vi "MaxIntenProj.vi"(10 "Dimension":u16, 11 "3D Array":u16[][][](array[numeric])) -> (3 "MaxProj":u16[][](array[numeric]))   [LabVIEW 2015]
panel:
  out "Intensity Graph":u16[][](graph)
  out "before size":i32[](array[numeric])
  out "size(s)":i32[](array[numeric])
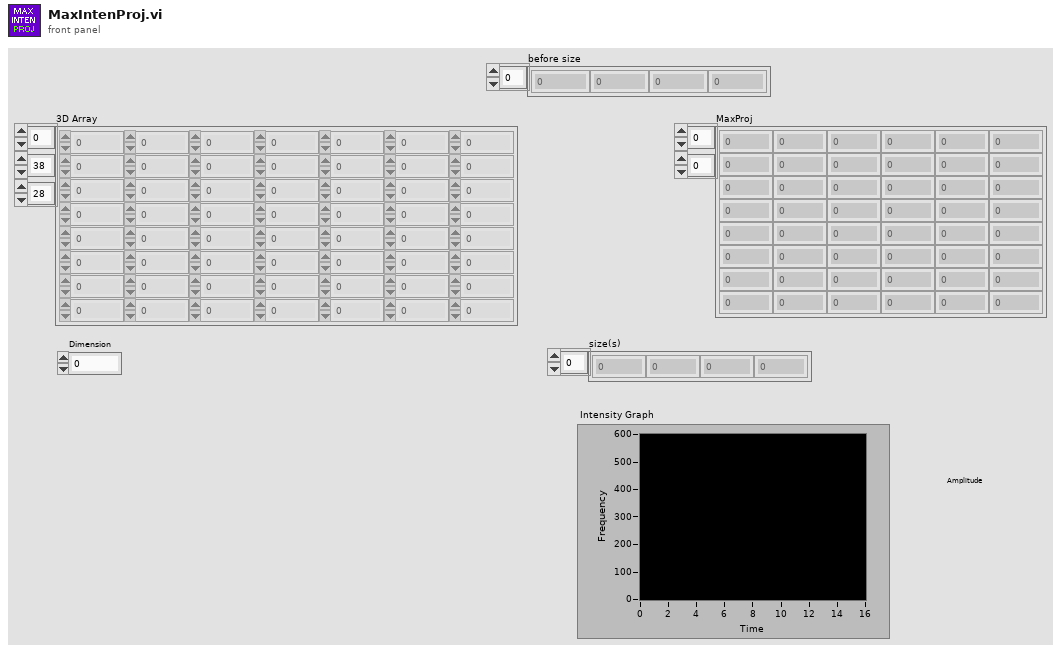
[diagram p1: front panel]
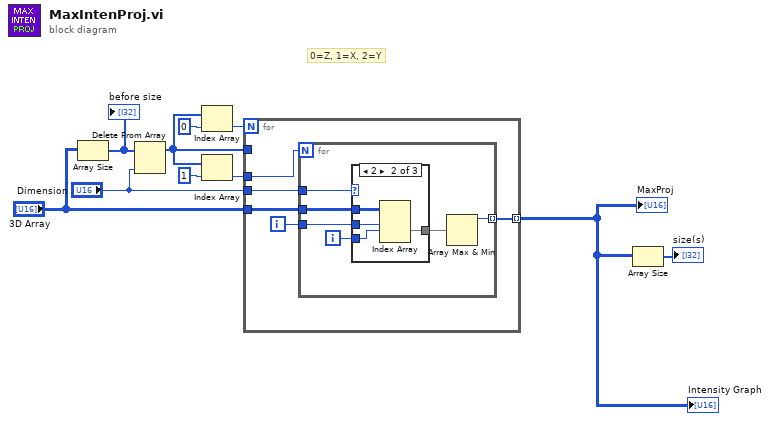
[diagram p0: block diagram]
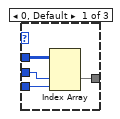
[diagram p2: hidden frame]
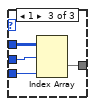
[diagram p3: hidden frame]
diagram:
  # "0=Z, 1=X, 2=Y"
  n1 = Array Size(array="3D Array") -> (size(s)=w10:i32[])
  "before size" <- w10
  n2 = Delete From Array(array=w10, index="Dimension") -> (array with subset deleted=w5:i32[])  [unwired: 1 in, 1 out]
  n3 = Index Array(array=w5, index=0) -> (element=w1:i32)
  n4 = Index Array(array=w5, index=1) -> (element=w4:i32)
  n5 = for {
    N: w1 -> [_]
    tunnel: w5 -> [_]
    tunnel: "3D Array" -> [w14]
    tunnel: "Dimension" -> [w13]
    tunnel: w4 -> [w12]
    tunnel: [w11] -> w2 mode=indexing
    i -> [w15]
    n6 = for {
      N: w12 -> [_]
      tunnel: w15 -> [w20]
      tunnel: w14 -> [w18]
      tunnel: w13 -> [w21]
      tunnel: [w16] -> w11 mode=indexing
      i -> [w19]
      n7 = case shown="2" w21 {
        tunnel: w19 -> [w22 w26 w30]
        tunnel: w20 -> [w23 w27 w33]
        tunnel: [w24 w28 w32] -> w17
        tunnel: w18 -> [w25 w29 w31]
        frame 0, Default {
          n8 = Index Array(array=w25, index (dim 1)=w23, index (dim 2)=w22) -> (element=w24:u16[])  [unwired: 1 in]
        }
        frame 2 {
          n9 = Index Array(array=w29, index (dim 0)=w27, index (dim 1)=w26) -> (element=w28:u16[])  [unwired: 1 in]
        }
        frame 1 {
          n10 = Index Array(array=w31, index (dim 0)=w33, index (dim 2)=w30) -> (element=w32:u16[])  [unwired: 1 in]
        }
      }
      n11 = Array Max & Min(array=w17) -> (max value=w16:u16)  [unwired: 3 out]
    }
  }
  "MaxProj" <- w2
  "Intensity Graph" <- w2
  n12 = Array Size(array=w2) -> (size(s)=→"size(s)":i32[])
